vi "Global_Device_IDs.vi"() -> ()   [LabVIEW 2017]
uses:
  TypeDef/CLUSTER_Arm_Device_IDs.ctl
  TypeDef/CLUSTER_Talon_Setup.ctl
  System Drivers/Phoenix-LabVIEW/Motor Controller/Controls/CTRE_Phoenix_MotorControl_FeedbackDevice.ctl
  TypeDef/CLUSTER_PID.ctl
  TypeDef/CLUSTER_Claw_Setup.ctl
  TypeDef/CLUSTER_Solonoid_Setup.ctl
  <vilib>/Rock Robotics/WPI/Solenoid/WPI_SolenoidChannel.ctl
panel:
  in  "Claw Setup":T1={"Left Solenoid"={"Pneumatics Control Module (0)"=0, "Solenoid Channel"=enum."Solenoid 0"}, "Right Solenoid"={"Pneumatics Control Module (0)"=0, "Solenoid Channel"=enum."Solenoid 0"}, "Left Talon Setup"={"Talon SRX ID"=0, "PhaseSensor"=FALSE, "Invert Motor?"=FALSE, "Phoenix Feedback Select"=-1, "pidLoopldx"=0, "PID"={"P"=0.0, "I"=0.0, "D"=0.0, "F"=0.0, "I Zone"=0.0}}, "Right Talon Setup"={"Talon SRX ID"=0, "PhaseSensor"=FALSE, "Invert Motor?"=FALSE, "Phoenix Feedback Select"=-1, "pidLoopldx"=0, "PID"={"P"=0.0, "I"=0.0, "D"=0.0, "F"=0.0, "I Zone"=0.0}}} {"Right Talon Setup"."Feedback Device" items=["None"=-1, "QuadEncoder"=0, "Analog"=2, "Tachometer"=4, "Pulse Width Encoded Position"=8, "Sensor Sum (S0 + S1)"=9, "Sensor Difference (D0 - D1)"=10, "Remote Source 0"=11, "Remote Source 1"=12, "Software Emulated"=15]; "Left Talon Setup"."Feedback Device" items=["None"=-1, "QuadEncoder"=0, "Analog"=2, "Tachometer"=4, "Pulse Width Encoded Position"=8, "Sensor Sum (S0 + S1)"=9, "Sensor Difference (D0 - D1)"=10, "Remote Source 0"=11, "Remote Source 1"=12, "Software Emulated"=15]}
  in  "Arm Setup":T7={"Elbow Setup"={"Talon SRX ID"=0, "PhaseSensor"=FALSE, "Invert Motor?"=FALSE, "Phoenix Feedback Select"=2, "pidLoopldx"=0, "PID"={"P"=0.0, "I"=0.0, "D"=0.0, "F"=0.0, "I Zone"=0.0}}, "Telescope Setup"={"Talon SRX ID"=0, "PhaseSensor"=FALSE, "Invert Motor?"=FALSE, "Phoenix Feedback Select"=-1, "pidLoopldx"=0, "PID"={"P"=0.0, "I"=0.0, "D"=0.0, "F"=0.0, "I Zone"=0.0}}, "Elbow Slave Setup"={"Talon SRX ID"=0, "PhaseSensor"=FALSE, "Invert Motor?"=FALSE, "Phoenix Feedback Select"=-1, "pidLoopldx"=0, "PID"={"P"=0.0, "I"=0.0, "D"=0.0, "F"=0.0, "I Zone"=0.0}}, "Telescope Slave Setup"={"Talon SRX ID"=0, "PhaseSensor"=FALSE, "Invert Motor?"=FALSE, "Phoenix Feedback Select"=-1, "pidLoopldx"=0, "PID"={"P"=0.0, "I"=0.0, "D"=0.0, "F"=0.0, "I Zone"=0.0}}} {"Telescope Slave Setup"."Feedback Device" items=["None"=-1, "QuadEncoder"=0, "Analog"=2, "Tachometer"=4, "Pulse Width Encoded Position"=8, "Sensor Sum (S0 + S1)"=9, "Sensor Difference (D0 - D1)"=10, "Remote Source 0"=11, "Remote Source 1"=12, "Software Emulated"=15]; "Elbow Slave Setup"."Feedback Device" items=["None"=-1, "QuadEncoder"=0, "Analog"=2, "Tachometer"=4, "Pulse Width Encoded Position"=8, "Sensor Sum (S0 + S1)"=9, "Sensor Difference (D0 - D1)"=10, "Remote Source 0"=11, "Remote Source 1"=12, "Software Emulated"=15]; "Telescope Setup"."Feedback Device" items=["None"=-1, "QuadEncoder"=0, "Analog"=2, "Tachometer"=4, "Pulse Width Encoded Position"=8, "Sensor Sum (S0 + S1)"=9, "Sensor Difference (D0 - D1)"=10, "Remote Source 0"=11, "Remote Source 1"=12, "Software Emulated"=15]; "Elbow Setup"."Feedback Device" items=["None"=-1, "QuadEncoder"=0, "Analog"=2, "Tachometer"=4, "Pulse Width Encoded Position"=8, "Sensor Sum (S0 + S1)"=9, "Sensor Difference (D0 - D1)"=10, "Remote Source 0"=11, "Remote Source 1"=12, "Software Emulated"=15]}
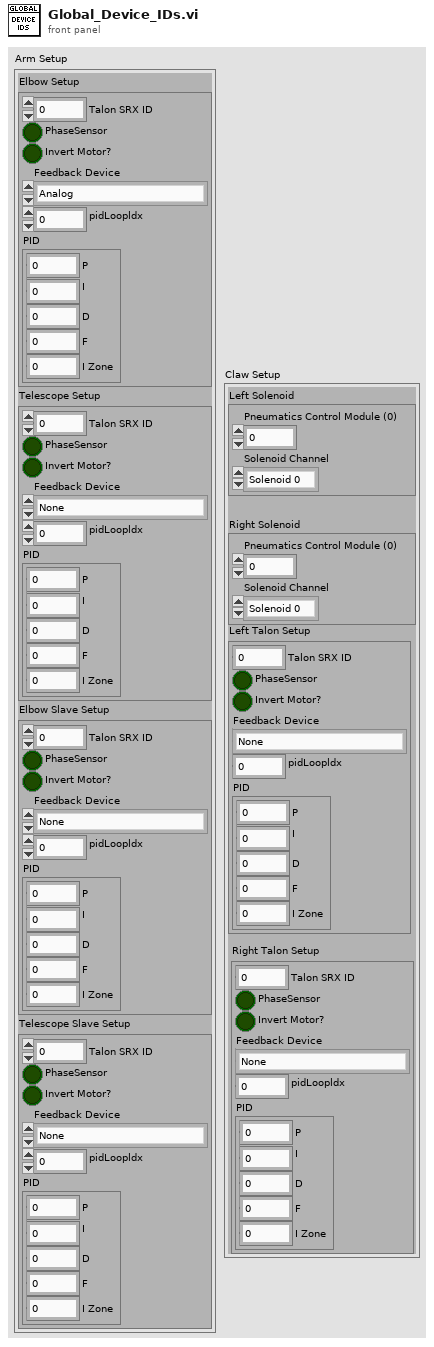
[diagram p1: front panel]
types:
  T1 = typedef "CLUSTER_Claw_Setup.ctl" = cluster{"Left Solenoid":T2, "Right Solenoid":T2, "Left Talon Setup":T4, "Right Talon Setup":T4}
  T2 = typedef "CLUSTER_Solonoid_Setup.ctl" = cluster{"Pneumatics Control Module (0)":u8, "Solenoid Channel":T3}
  T3 = typedef "WPI_SolenoidChannel.ctl" = enum8{"Solenoid 0", "Solenoid 1", "Solenoid 2", "Solenoid 3", "Solenoid 4", "Solenoid 5", "Solenoid 6", "Solenoid 7", "Invalid"}
  T4 = typedef "CLUSTER_Talon_Setup.ctl" = cluster{"Talon SRX ID":u8, "PhaseSensor":bool, "Invert Motor?":bool, "Phoenix Feedback Select":T5, "pidLoopldx":i32, "PID":T6}
  T5 = typedef "CTRE_Phoenix_MotorControl_FeedbackDevice.ctl" = i8
  T6 = typedef "CLUSTER_PID.ctl" = cluster{"P":dbl, "I":dbl, "D":dbl, "F":dbl, "I Zone":dbl}
  T7 = typedef "CLUSTER_Arm_Device_IDs.ctl" = cluster{"Elbow Setup":T4, "Telescope Setup":T4, "Elbow Slave Setup":T4, "Telescope Slave Setup":T4}
diagram:
